vi "solar_msg UE Destroy.vi"(8 "error in (no error)":errorcluster, 11 "UserEvent":refnum<user-event>) -> (0 "error out":errorcluster)   [LabVIEW 2018]
doc: "This destroys a <b>User Event</b> reference."
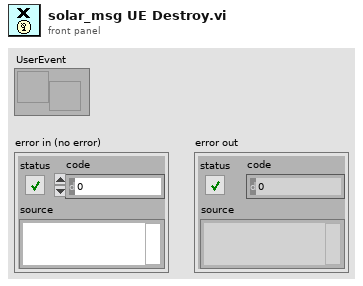
[diagram p1: front panel]
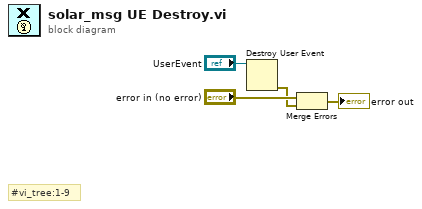
[diagram p0: block diagram]
diagram:
  # "#vi_tree:1-9"
  n1 = Destroy User Event(user event="UserEvent") -> (error out=w1:errorcluster)  [unwired: 1 in]
  n2 = Merge Errors("error in (no error)", w1) -> (→"error out":errorcluster)
